vi "CheckForChange.vi"(10 "Original Settings":T1={"Name of test"="", "Date"=timestamp(0 s since 1904-01-01), "Location"="", "Template"="", "Soundcard"="", "resolution"=0, "Sampling rate"=0, "Ch1 Gain "=0.0, "Ch2 Gain"=0.0, "Sample time (s)"=0.0, "Pre-trigger (s)"=0.0, "Hammer Threshold"=0.0, "Positions"=0, "Taps/Position"=0, "Set Names"="", "Freq resolution"=0.0, "Hammer cutoff"=0.0, "Mic cutoff"=0.0, "Double bounce "=0.0, "Hammer Cal"=0.0, "dB Offset"=0.0, "Accel Cal"=0.0, "Vibrometer Cal"=0.0, "Mic Cal"=0.0, "Output"=0, "Voltage Cal"=0.0, "Vibrometer Port"="", "Range"=0, "High Pass"=0, "Bandwidth"=0, "X Range"=[], "Y Range"=[], "dB Spread"=0.0, "Trigger"=0, "Ch_1"=0, "Ch_2"=0, "flip?"=FALSE, "60Hz"=FALSE, "Time offset"=0.0, "Piezo Cal"=1.0, "Default Notes"=""} {"Ch_2" min=1 step=1; "Ch_1" min=1 max=100 step=1; "Trigger" items=["Hammer (force)", "Self-tap", "Spacebar"]; "Bandwidth" items=["1 kHz"=1, "5 kHz"=5, "10 kHz"=10, "25 kHz"=25, "50 kHz"=50, "100 kHz"=100]; "High Pass" items=["Off", "13 Hz", "104 Hz"]; "Range" items=["10 mm/s"=1, "20 mm/s"=2, "50 mm/s"=5, "100 mm/s"=10, "200 mm/s"=20, "500 mm/s"=50, "1 m/s"=100, "2 m/s"=200]; "Output" items=["Accelerometer", "Speed (from acceleration)", "Microphone", "Vibrometer", "Piezo"]; "Voltage Cal" format="%#_13g"; "Ch2 Gain" format="%#_13g"; "Ch1 Gain" format="%#_13g"; "Double bounce" min=0.0; "Mic cutoff" min=0.0 format="%#_4g"; "Hammer cutoff" min=0.0 format="%#_4g"; "Freq resolution" min=0.0; "Pre-trigger (s)" format="%#_13g"; "Date" format="%<%H:%M\n%d/%m/%y>T"; "resolution" items=["16 bit"=16, "24 bit"=24, "32 bit"=32]; "Sampling rate" items=["22050 samp/s"=22050, "44100 samp/s"=44100, "48000 samp/s"=48000]}, 11 "Current Settings":T1={"Name of test"="", "Date"=timestamp(0 s since 1904-01-01), "Location"="", "Template"="", "Soundcard"="", "resolution"=0, "Sampling rate"=0, "Ch1 Gain "=0.0, "Ch2 Gain"=0.0, "Sample time (s)"=0.0, "Pre-trigger (s)"=0.0, "Hammer Threshold"=0.0, "Positions"=0, "Taps/Position"=0, "Set Names"="", "Freq resolution"=0.0, "Hammer cutoff"=0.0, "Mic cutoff"=0.0, "Double bounce "=0.0, "Hammer Cal"=0.0, "dB Offset"=0.0, "Accel Cal"=0.0, "Vibrometer Cal"=0.0, "Mic Cal"=0.0, "Output"=0, "Voltage Cal"=0.0, "Vibrometer Port"="", "Range"=0, "High Pass"=0, "Bandwidth"=0, "X Range"=[], "Y Range"=[], "dB Spread"=0.0, "Trigger"=0, "Ch_1"=0, "Ch_2"=0, "flip?"=FALSE, "60Hz"=FALSE, "Time offset"=0.0, "Piezo Cal"=1.0, "Default Notes"=""} {"Ch_2" min=1 step=1; "Ch_1" min=1 max=100 step=1; "Trigger" items=["Hammer (force)", "Self-tap", "Spacebar"]; "Bandwidth" items=["1 kHz"=1, "5 kHz"=5, "10 kHz"=10, "25 kHz"=25, "50 kHz"=50, "100 kHz"=100]; "High Pass" items=["Off", "13 Hz", "104 Hz"]; "Range" items=["10 mm/s"=1, "20 mm/s"=2, "50 mm/s"=5, "100 mm/s"=10, "200 mm/s"=20, "500 mm/s"=50, "1 m/s"=100, "2 m/s"=200]; "Output" items=["Accelerometer", "Speed (from acceleration)", "Microphone", "Vibrometer", "Piezo"]; "Voltage Cal" format="%#_13g"; "Ch2 Gain" format="%#_13g"; "Ch1 Gain" format="%#_13g"; "Double bounce" min=0.0; "Mic cutoff" min=0.0 format="%#_4g"; "Hammer cutoff" min=0.0 format="%#_4g"; "Freq resolution" min=0.0; "Pre-trigger (s)" format="%#_13g"; "Date" format="%<%H:%M\n%d/%m/%y>T"; "resolution" items=["16 bit"=16, "24 bit"=24, "32 bit"=32]; "Sampling rate" items=["22050 samp/s"=22050, "44100 samp/s"=44100, "48000 samp/s"=48000]}) -> (2 "change?":bool, 3 "list of changes":string)   [LabVIEW 2022 SP3]
uses:
  PreferencesControl.ctl
  <vilib>/Utility/error.llb/Trim Whitespace One-Sided.vi
panel:
  # "Hz"
  # "dB"
  # "dB"
  # "sec"
  # "sec"
  # "mV/Pa"
  # "mV/m/s2"
  # "mV/mm/s"
  # "V/N"
  # "sec"
  # "sec"
  # "mV/N"
  # "a.u."
  # "a.u."
  # "sec"
  # "Hz"
  # "dB"
  # "dB"
  # "sec"
  # "sec"
  # "mV/Pa"
  # "mV/m/s2"
  # "mV/mm/s"
  # "V/N"
  # "sec"
  # "sec"
  # "mV/N"
  # "a.u."
  # "a.u."
  # "sec"
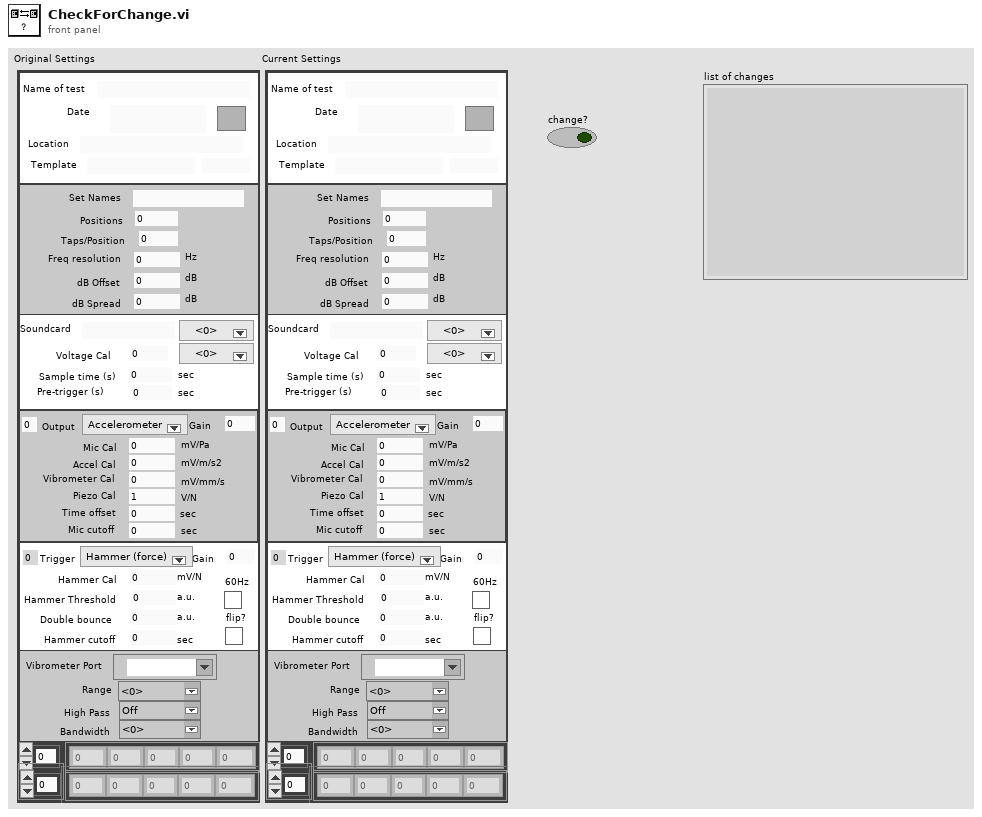
[diagram p1: front panel]
types:
  T1 = typedef "PreferencesControl.ctl" = cluster{"Name of test":string, "Date":timestamp, "Location":string, "Template":string, "Soundcard":string, "resolution":u16, "Sampling rate":u16, "Ch1 Gain ":dbl, "Ch2 Gain":dbl, "Sample time (s)":dbl, "Pre-trigger (s)":dbl, "Hammer Threshold":dbl, "Positions":i16, "Taps/Position":i16, "Set Names":string, "Freq resolution":dbl, "Hammer cutoff":dbl, "Mic cutoff":dbl, "Double bounce ":dbl, "Hammer Cal":dbl, "dB Offset":dbl, "Accel Cal":dbl, "Vibrometer Cal":dbl, "Mic Cal":dbl, "Output":u16, "Voltage Cal":dbl, "Vibrometer Port":refnum<visa-resource-name>, "Range":u16, "High Pass":u16, "Bandwidth":u16, "X Range":cluster{"Minimum":dbl, "Maximum":dbl, "Increment":dbl, "Minor Increment":dbl, "Start":dbl}[], "Y Range":cluster{"Minimum":dbl, "Maximum":dbl, "Increment":dbl, "Minor Increment":dbl, "Start":dbl}[], "dB Spread":dbl, "Trigger":u16, "Ch_1":u8, "Ch_2":u8, "flip?":bool, "60Hz":bool, "Time offset":dbl, "Piezo Cal":dbl, "Default Notes":string}
  T2 = cluster{"Name of test":bool, "Date":bool, "Location":bool, "Template":bool, "Soundcard":bool, "resolution":bool, "Sampling rate":bool, "Ch1 Gain ":bool, "Ch2 Gain":bool, "Sample time (s)":bool, "Pre-trigger (s)":bool, "Hammer Threshold":bool, "Positions":bool, "Taps/Position":bool, "Set Names":bool, "Freq resolution":bool, "Hammer cutoff":bool, "Mic cutoff":bool, "Double bounce ":bool, "Hammer Cal":bool, "dB Offset":bool, "Accel Cal":bool, "Vibrometer Cal":bool, "Mic Cal":bool, "Output":bool, "Voltage Cal":bool, "Vibrometer Port":bool, "Range":bool, "High Pass":bool, "Bandwidth":bool, "X Range":cluster{"Minimum":bool, "Maximum":bool, "Increment":bool, "Minor Increment":bool, "Start":bool}[], "Y Range":cluster{"Minimum":bool, "Maximum":bool, "Increment":bool, "Minor Increment":bool, "Start":bool}[], "dB Spread":bool, "Trigger":bool, "Ch_1":bool, "Ch_2":bool, "flip?":bool, "60Hz":bool, "Time offset":bool, "Piezo Cal":bool, "Default Notes":bool}
  T3 = cluster{"Minimum":bool, "Maximum":bool, "Increment":bool, "Minor Increment":bool, "Start":bool}[]
  T4 = cluster{"Minimum":bool, "Maximum":bool, "Increment":bool, "Minor Increment":bool, "Start":bool}
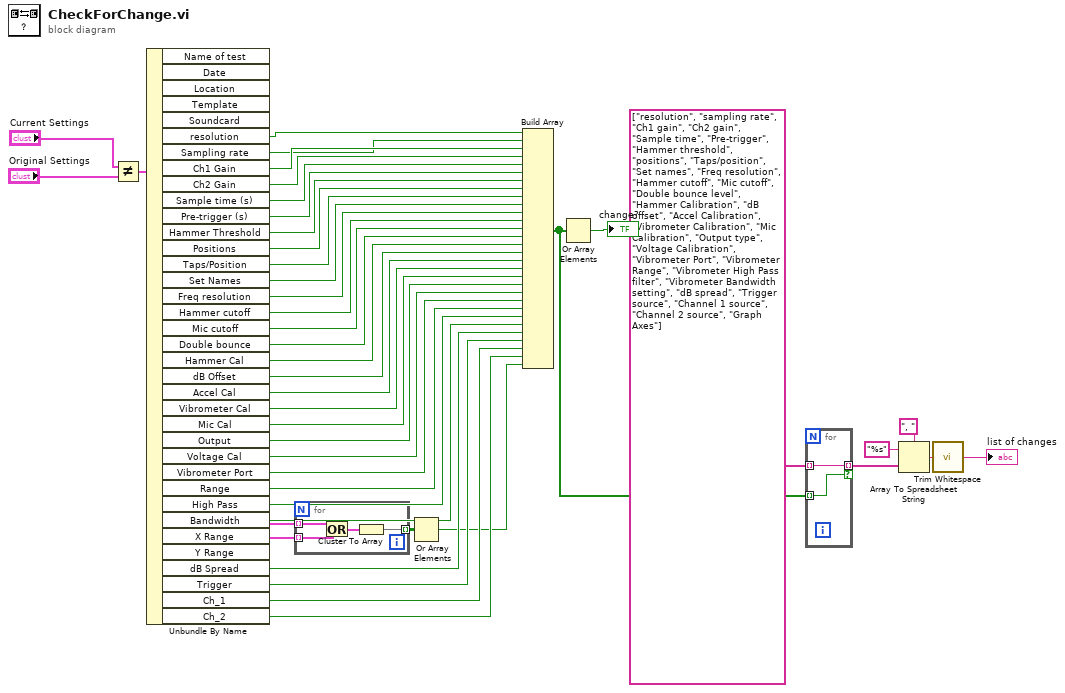
[diagram p0: block diagram]
diagram:
  n1 = Not Equal?(x="Current Settings", y="Original Settings") -> (x != y?=w7:T2)
  n2 = Unbundle By Name(w7) -> ("resolution"=w8:bool, "Sampling rate"=w9:bool, "Ch1 Gain"=w10:bool, "Ch2 Gain"=w11:bool, "Sample time (s)"=w12:bool, "Pre-trigger (s)"=w13:bool, "Hammer Threshold"=w14:bool, "Positions"=w15:bool, "Taps/Position"=w16:bool, "Set Names"=w17:bool, "Freq resolution"=w18:bool, "Hammer cutoff"=w19:bool, "Mic cutoff"=w20:bool, "Double bounce"=w21:bool, "Hammer Cal"=w22:bool, "dB Offset"=w23:bool, "Accel Cal"=w24:bool, "Vibrometer Cal"=w25:bool, "Mic Cal"=w26:bool, "Output"=w27:bool, "Voltage Cal"=w28:bool, "Vibrometer Port"=w29:bool, "Range"=w30:bool, "High Pass"=w31:bool, "Bandwidth"=w32:bool, "X Range"=w4:T3, "Y Range"=w3:T3, "dB Spread"=w33:bool, "Trigger"=w34:bool, "Ch_1"=w36:bool, "Ch_2"=w37:bool)  [unwired: 5 out]
  n3 = for {
    tunnel: w4 -> [w48] mode=indexing
    tunnel: w3 -> [w47] mode=indexing
    tunnel: [w45] -> w2 mode=indexing
    n4 = Or(x=w48, y=w47) -> (x .or. y?=w46:T4)
    n5 = Cluster To Array(cluster=w46) -> (array=w45:bool[])
  }
  n6 = Or Array Elements(Boolean array=w2) -> (logical OR=w1:bool)
  n7 = Build Array(w8, w9, w10, w11, w12, w13, w14, w15, w16, w17, w18, w19, w20, w21, w22, w23, w24, w25, w26, w27, w28, w29, w30, w31, w32, w33, w34, w36, w37, w1) -> (w38:bool[])
  n8 = Or Array Elements(Boolean array=w38) -> (logical OR=→"change?":bool)
  n9 = for {
    tunnel: w38 -> [w49] mode=indexing
    tunnel: string[] ["resolution", "sampling rate", "Ch1 gain", "Ch2 gain", "Sample time", "Pre-trigger", "Hammer threshold", "positions", "Taps/position", "Set names", "Freq resolution", "Hammer cutoff", "Mic cutoff", "Double bounce level", "Hammer Calibration", "dB offset", "Accel Calibration", "Vibrometer Calibration", "Mic Calibration", "Output type", "Voltage Calibration", "Vibrometer Port", "Vibrometer Range", "Vibrometer High Pass filter", "Vibrometer Bandwidth setting", "dB spread", "Trigger source", "Channel 1 source", "Channel 2 source", "Graph Axes"] -> [w50] mode=indexing
    tunnel: [w50] -> w40 mode=indexing if=w49
  }
  n10 = Array To Spreadsheet String(delimiter (Tab)=", ", array=w40, 3:"%s" ("format string")) -> (spreadsheet string=w43:string)
  n11 = call <vilib>:"Trim Whitespace.vi"("string"=w43) -> ("trimmed string"=→"list of changes":string)  [unwired: 1 in]
